vi "BooleanOneShot[1].vi"(0 "inpout array":bool[](array[boolean]), 1 "input":bool=TRUE) -> (2 "output array":bool[](array[boolean]), 3 "rising edge":bool=TRUE, 4 "falling edge":bool)   [LabVIEW 2019]
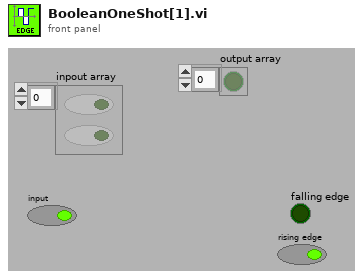
[diagram p1: front panel]
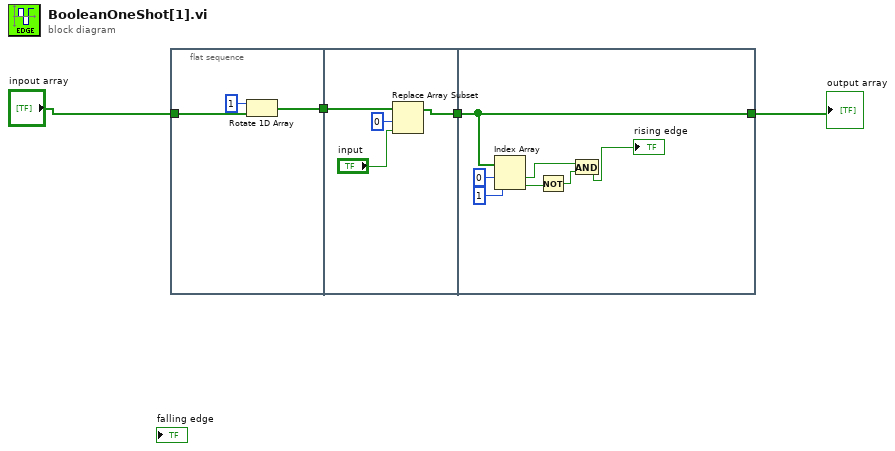
[diagram p0: block diagram]
diagram:
  n1 = flat-sequence {
    tunnel: "inpout array" -> [w7]
    tunnel: [w5] -> w4
    tunnel: w4 -> [w11]
    tunnel: [w8] -> w3
    tunnel: [w15] -> w1
    tunnel: w3 -> [w15]
    frame #0 {
      n2 = Rotate 1D Array(1:w7, 2:1 ("n")) -> (0:w5:bool[])
    }
    frame #1 {
      n3 = Replace Array Subset(array=w11, new element="input", index=0) -> (w8:bool[])
    }
    frame #2 {
      n4 = Index Array(array=w15, index #1=0 ("index"), index #2=1 ("index")) -> (element #1=w12:bool, element #2=w14:bool)
      n5 = Not(x=w14) -> (.not. x?=w13:bool)
      n6 = And(x=w12, y=w13) -> (x .and. y?=→"rising edge":bool)
    }
  }
  "output array" <- w1
